vi "drawRoi.vi"(6 "Colors (Red)":u32[](array[colorbox])=[16711680], 8 "bit depth":enum16{"16bits", "14bits", "12bits", "8bits"}(ring), 9 "ROI":refnum<vi>, 10 "Reff image":T1, 11 "Whole image":T1) -> (0 "size":i32, 1 "mean":dbl, 2 "Reff image":T1(plugin-control), 3 "Image Out":T1, 4 "Percentile alert":bool)   [LabVIEW 2023]
uses:
  <vilib>/vision/Image Controls.llb/IMAQ Image.ctl
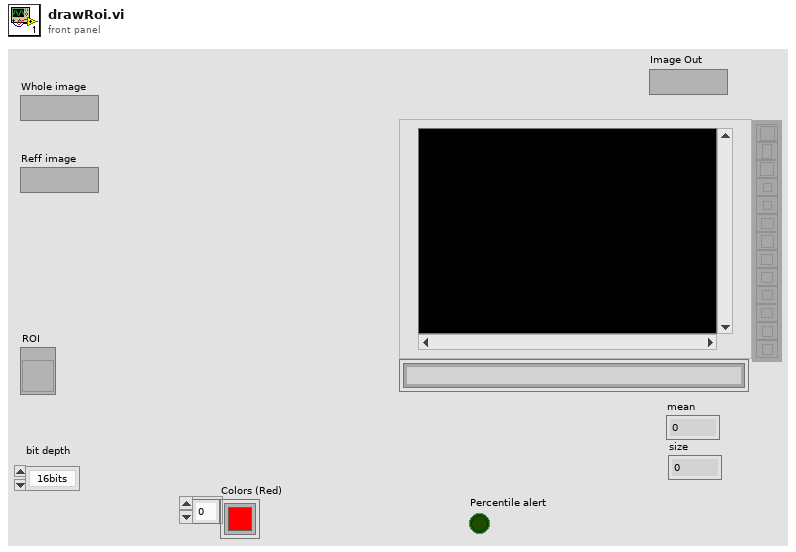
[diagram p1: front panel]
types:
  T1 = typedef "IMAQ Image.ctl" = refnum<image>
  T2 = cluster{"Global Rectangle":i32[], "Contours":cluster{"Contour Type":u32, "ROI Type":u32, "Points":i32[]}[]}
  T3 = cluster{"mean (ROI)":dbl, "max (ROI)":i16, "max_counts":dbl, "image_size":i32, "# Sat. Pixels":sgl, "# in percentile":dbl}
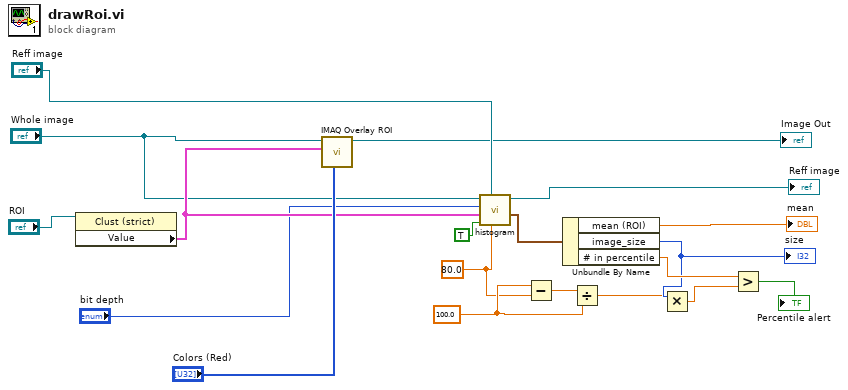
[diagram p0: block diagram]
diagram:
  w4 = 100.0 ("y")
  w3 = 80.0 ("Percentile check")
  n1 = property class="Clust (strict)"(reference="ROI") -> ("Value"=w17:T2)  [unwired: 1 in, 2 out]
  n2 = call "IMAQ Overlay ROI"("Colors (Green)"="Colors (Red)", "ROI Descriptor"=w17, "Image"="Whole image") -> ("Image Out"=→"Image Out":T1)  [unwired: 7 in, 1 out]
  n3 = call "histogram.vi"("Percentile check"=w3, "Image ROI"="Reff image", "useROI"=TRUE, "ROI Descriptor"=w17, "bit depth"="bit depth", "Image"="Whole image") -> ("Statistics"=w12:T3, "Image Out (ROI)"=→"Reff image":T1)  [unwired: 1 in, 3 out]
  n4 = Subtract(x=w4, y=w3) -> (x-y=w2:dbl)
  n5 = Unbundle By Name(w12) -> ("mean (ROI)"=→"mean":dbl, "image_size"=w6:i32, "# in percentile"=w8:dbl)
  "size" <- w6
  n6 = Divide(x=w2, y=w4) -> (x/y=w5:dbl)
  n7 = Multiply(x=w6, y=w5) -> (x*y=w7:dbl)
  n8 = Greater?(x=w8, y=w7) -> (0:→"Percentile alert":bool)
